vi "OL_WaveSaver_fpga.vi"() -> ()   [LabVIEW 2020]
uses:
  <vilib>/rvi/Emulation/niFpgaGetClockAttributes.vi
  <vilib>/rvi/Emulation/niFpgaSctlEmulationGetInTimedLoop.vi
  <vilib>/rvi/Emulation/niFpgaEmulationReportErrorSimple.vi
  <vilib>/rvi/eio/common/nirviEmuTemplateMethod_errors.vi
  <vilib>/rvi/interface/RandomDataEmulation/nirviRandomDataMultiElementFPGAFIFO.vi
  <instcachedir>/0/nirviRandomDataMultiElementFPGAFIFO_3E9965BA1FAD4E7B8DABA31768A09B1F.lvgen/nirviRandomDataMultiElementFPGAFIFO_3E9965BA1FAD4E7B8DABA31768A09B1F_001.vi
  <vilib>/rvi/interface/RandomDataEmulation/niFpgaRandomDataHandleErrors.vi
  <vilib>/rvi/Emulation/niFpgaCriticalErrorInLSC.vi
  <vilib>/eio/EIONode/EIONode.xnode
  <vilib>/rvi/DataTransferAndStorage/Container/XNode/niFpgaContainer.xnode
  <vilib>/rvi/interface/RandomDataEmulation/nirviRandomDataFpgaMultiElementTemplate.vi
panel:
  in  "decimation":i16
  in  "stop":bool
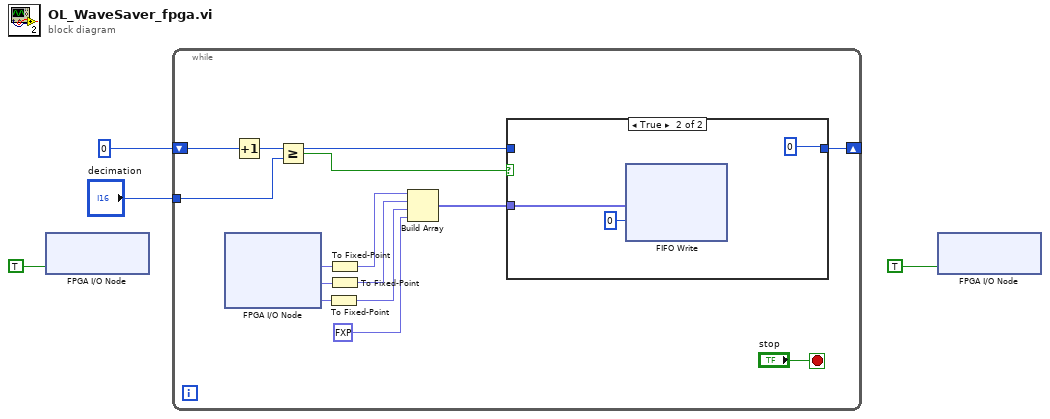
[diagram p0: block diagram]
diagram:
  n1 = xnode "FPGA I/O Node"("Mod1/Start"=TRUE ("Mod2/Start")) -> ()  [unwired: 2 in, 2 out]
  n2 = while {
    shift-right: [w13] -> _
    shift-left: i16 0 -> [w17]
    tunnel: "decimation" -> [w16]
    stop <- "stop" stop-if-true
    n3 = xnode "FPGA I/O Node"() -> ("Mod1/AI0"=w11:fxp<+/-,24,5>, "Mod1/AI1"=w10:fxp<+/-,24,5>, "Mod1/AI2"=w9:fxp<+/-,24,5>)  [unwired: 4 in, 4 out]
    n4 = Increment(x=w17) -> (x+1=w14:i16)
    n5 = Greater Or Equal?(x=w14, y=w16) -> (x >= y?=w15:bool)
    n6 = To Fixed-Point(number=w9) -> (fixed-point=w6:fxp<+/-,64,20>)  [unwired: 1 in]
    n7 = To Fixed-Point(number=w11) -> (fixed-point=w8:fxp<+/-,64,20>)  [unwired: 1 in]
    n8 = To Fixed-Point(number=w10) -> (fixed-point=w7:fxp<+/-,64,20>)  [unwired: 1 in]
    n9 = Build Array(w8, w7, w6, fxp<+/-,64,20> 0.0 ("element")) -> (w12:fxp<+/-,64,20>[])
    n10 = case shown="True" w15 {
      tunnel: w14 -> [w19 _]
      tunnel: [w19 i16 0] -> w13
      tunnel: w12 -> [_ w20]
      frame False {
      }
      frame True {
        n11 = xnode ("FIFO Write")("Element"=w20, "Timeout"=0) -> ()  [unwired: 1 in, 2 out]
      }
    }
  }
  n12 = xnode "FPGA I/O Node"("Mod1/Stop"=TRUE ("Mod2/Stop")) -> ()  [unwired: 2 in, 2 out]
